vi "PH_Sequencer.get Head Attributes.vi"(2 "PowerUnit":T1=enum."MA-FR", 3 "Heads":T2[](array[typedef]) {"Information"."State" items=["no info", "off/false/out", "on/true/in", "Failure", "Alarm", "Status 1", "Status 2", "Status 3"]}) -> (0 "Head":T2={"PowerUnit"=enum."no Info", "GUI Ref"=refnum, "Information"={"State"=2, "Waiting Time [s]"=1800.0, "PU State SM"=enum.".", "PU Timeout SM"=enum."."}, "linked?"=FALSE, "GUI Ref Current Voltage"=refnum} {"Information"."State" items=["no info", "off/false/out", "on/true/in", "Failure", "Alarm", "Status 1", "Status 2", "Status 3"]}, 1 "Head found?":bool)   [LabVIEW 2014, in "PH_Sequencer.lvlib"]
doc: "This VI searches head attributes."
uses:
  PH_Sequencer.lvlib
  PH_Sequencer.Head.ctl
  PH_PP_Common/PH_PP_Common.PUs.ctl
  PH_Sequencer.PU Information for GUI.ctl
  PH_StatusHandler/PH_StatusHandler.GUI element.ctl
  PH_PowerUnit_BaseClass/PH_PowerUnit_BaseClass.SM States.ctl
  PH_Sequencer.PU Information.ctl
  PH_StatusHandler/PH_StatusHandler.Status.ctl
  PH_PP_Common/PH_PP_Common.lvlib
  PH_StatusHandler/PH_StatusHandler.lvlib
  PH_PowerUnit_BaseClass/PH_PowerUnit_BaseClass.lvlib
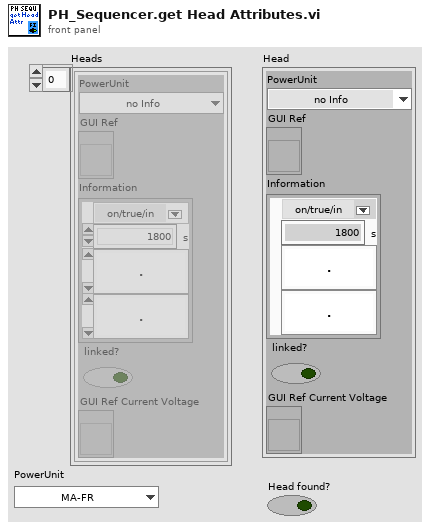
[diagram p1: front panel]
types:
  T1 = typedef "PH_PP_Common.lvlib/PH_PP_Common.PUs.ctl" = enum16{"no Info", "PA-19mm-1", "PA-19mm-2", "PA-45mm-PILC", "PA-45mm-MAIN", "MA-PU-1", "MA-PU-2", "MA-PU-3", "MA-PU-4", "MA-PU-5", "MA-PU-6", "MA-FR", "MA-PILC", "PA-45mm-DP"}
  T2 = typedef "PH_Sequencer.lvlib/PH_Sequencer.Head.ctl" = cluster{"PowerUnit":T1, "GUI Ref":refnum<vi>, "Information":T3, "linked?":bool, "GUI Ref Current Voltage":refnum<vi>}
  T3 = typedef "PH_Sequencer.lvlib/PH_Sequencer.PU Information.ctl" = cluster{"State":T4, "Waiting Time [s]":dbl, "PU State SM":T5, "PU Timeout SM":T5}
  T4 = typedef "PH_StatusHandler.lvlib/PH_StatusHandler.Status.ctl" = i16
  T5 = typedef "PH_PowerUnit_BaseClass.lvlib/PH_PowerUnit_BaseClass.SM States.ctl" = enum16{".", "Stand by", "Switch PU on", "Configure", "Set Default Voltage", "Set STANDBY", "Set READY", "Wait for Shot Cmd", "Open Dump Rods", "Open Ross Relais", "Close Ross Relais", "Switch PSU on", "Switch PSU off", "Charge", "Switch GD Channel on", "Close Dump Rods", "Rods-TO", "RR-TO", "PSU-TO", "Trigger-TO"}
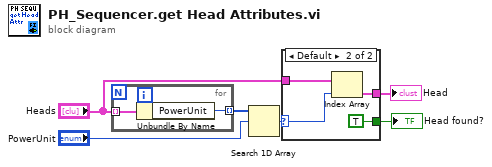
[diagram p0: block diagram]
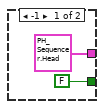
[diagram p2: hidden frame]
diagram:
  n1 = for {
    tunnel: "Heads" -> [w8] mode=indexing
    tunnel: [w7] -> w1 mode=indexing
    n2 = Unbundle By Name(w8) -> ("PowerUnit"=w7:T1)
  }
  n3 = Search 1D Array(1D array=w1, element="PowerUnit") -> (index of element=w3:i32)  [unwired: 1 in]
  n4 = case shown="Default" w3 {
    selector: w3 -> [_ w14]
    tunnel: "Heads" -> [_ w13]
    tunnel: [T2 {"PowerUnit"=enum."no Info", "GUI Ref"=refnum, "Information"={"State"=0, "Waiting Time [s]"=0.0, "PU State SM"=enum.".", "PU Timeout SM"=enum."."}, "linked?"=FALSE, "GUI Ref Current Voltage"=refnum} ("Head") w12] -> w5
    tunnel: [FALSE TRUE] -> w6
    frame -1 {
    }
    frame Default {
      n5 = Index Array(array=w13, index=w14) -> (element=w12:T2)
    }
  }
  "Head found?" <- w6
  "Head" <- w5
